vi "Read Temperature.vi"(8 "error in (no error)":errorcluster, 11 "Thermometer Base in":refnum<class "Thermometer Base.lvclass">) -> (0 "error out":errorcluster, 2 "Temperature":dbl format="%#_g °C", 3 "Thermometer Base out":refnum<class "Thermometer Base.lvclass">)   [LabVIEW 2023, in "Thermometer.lvlib" / "Thermometer Base.lvlib" / "Thermometer Base.lvclass"]
uses:
  Thermometer Base.lvclass
  Interfaces/IConfigure Thermometer/IConfigure Thermometer.lvclass
  Thermometer Base.lvclass/Thermometer Base.ctl
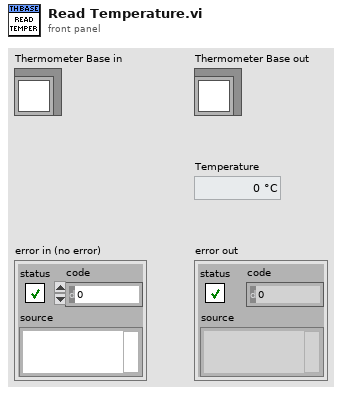
[diagram p1: front panel]
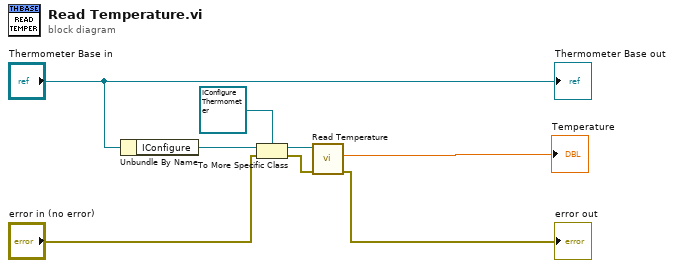
[diagram p0: block diagram]
diagram:
  n1 = Unbundle By Name("Thermometer Base in") -> ("IConfigure"=w6:refnum<class "IConfigure.lvclass">)
  n2 = To More Specific Class(target class=refnum<class "IConfigure Thermometer.lvclass"> refnum ("HAL Interfaces.lvlib:IConfigure Thermometer.lvclass"), reference=w6, error in="error in (no error)") -> (specific class reference=w8:refnum<class "IConfigure Thermometer.lvclass">, error out=w7:errorcluster)
  n3 = call-dynamic "Read Temperature.vi"("error in (no error)"=w7, "IConfigure Thermometer in"=w8) -> ("error out"=→"error out":errorcluster, "Temperature"=→"Temperature":dbl)  [unwired: 7 in, 1 out]
  "Thermometer Base out" <- "Thermometer Base in"
